vi "PAXStop.vi"(2 "error in":errorcluster caption="error in (no error)" {"code" format="%.0x"}, 3 "VISA 输入":refnum<visa-resource-name> caption="instrument handle") -> (0 "error out":errorcluster)   [LabVIEW 2018]
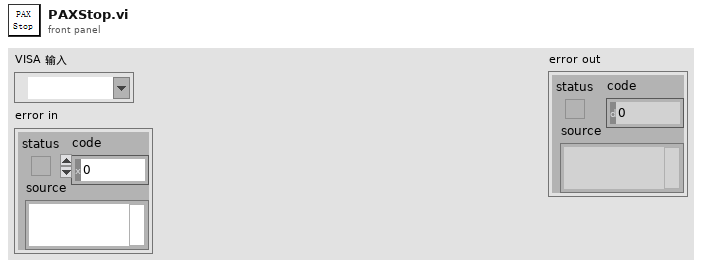
[diagram p1: front panel]
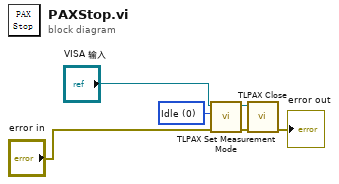
[diagram p0: block diagram]
diagram:
  w6 = 0 items=["Idle", "Half Waveplate Rotation - 512 Point FFT", "Half Waveplate Rotation - 1024 Point FFT", "Half Waveplate Rotation - 2048 Point FFT", "Full Waveplate Rotation - 512 Point FFT", "Full Waveplate Rotation - 1024 Point FFT", "Full Waveplate Rotation - 2048 Point FFT", "Double Waveplate Rotation - 512 Point FFT", "Double Waveplate Rotation - 1024 Point FFT", "Double Waveplate Rotation - 2048 Point FFT"] ("Mode (Double Waveplate Rotation - 2048 Point FFT)")
  n1 = call <instrlib>:"TLPAX Set Measurement Mode.vi"("error in (no error)"="error in", "Mode (Double Waveplate Rotation - 2048 Point FFT)"=w6, "instrument handle"="VISA 输入") -> ("error out"=w4:errorcluster, "instrument handle out"=w5:refnum<visa-resource-name>)  [unwired: 7 in]
  n2 = call <instrlib>:"TLPAX Close.vi"("error in (no error)"=w4, "instrument handle"=w5) -> ("error out"=→"error out":errorcluster)  [unwired: 9 in]
